vi "Scripted Autonomous.vi"   [LabVIEW 2015]
uses:
  Common Code/Change Detect Int.vi
  Robot Global Data.vi
types:
  T1 = typedef "Auton Command Cluster.ctl" = cluster{"Command ID":i32, "maxTime":dbl, "Y Distance":dbl, "Heading":dbl, "Throttle":dbl, "Async":dbl, "Velocity":dbl, "Acceleration":dbl, "To":dbl, "Condition":dbl, "Shot Type":dbl, "Left RPM":dbl, "Override RPM":i32, "Override Angle":i32, "Right RPM":dbl, "Angle":dbl, "Intake Mode":i32, "Intake Cmd":i32, "Intake O":i32, "Eject O":i32, "Angle O":i32, "Arm O":i32, "Intake Speed":dbl, "Eject Speed":dbl, "Arm Angle":dbl, "Arm Speed":dbl, "Intake?":i32, "Eject?":i32}
  T2 = typedef "Drivetrain Status Cluster.ctl" = cluster{"Modes":T3, "Y (Throttle)":dbl, "X (Steer)":dbl, "Gyro In Range?":bool, "Distance Drive Finished?":bool, "Stop Eject Lockout":bool, "Dist Drive Status":T4, "Y Target":dbl, "Heading Target":dbl, "Vision Target Aligned?":bool, "Gear":dbl, "1st Gear Time":dbl, "2nd Gear Time":dbl, "1st Gear Shifts":dbl, "2nd Gear Shifts":dbl}
  T3 = typedef "Drivetrain Modes.ctl" = enum16{"Climb", "Manual", "Ball Vision Targeting", "Goal Vision Targeting", "PID Distance Drive", "Hybrid"}
  T4 = typedef "Dist Drive Status.ctl" = cluster{"Y In Range":bool, "X In Range":bool, "Gyro In Range":bool, "Y Dist":dbl, "X Dist":dbl, "Gyro":dbl}
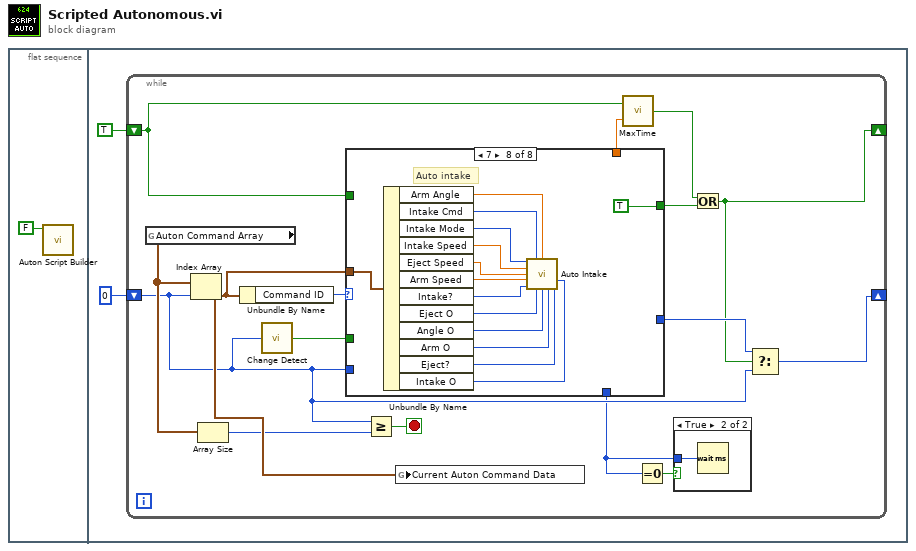
[diagram p0: block diagram]
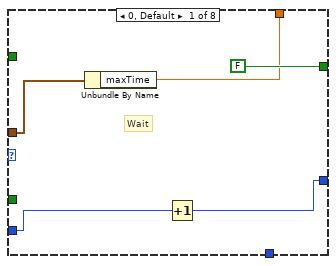
[diagram p3: hidden frame]
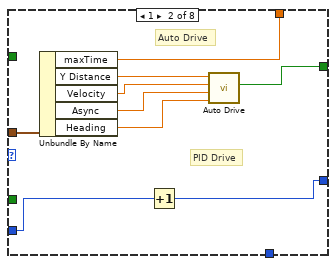
[diagram p4: hidden frame]
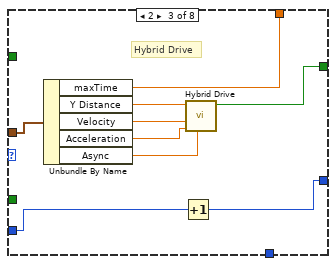
[diagram p5: hidden frame]
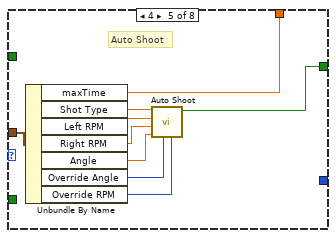
[diagram p7: hidden frame]
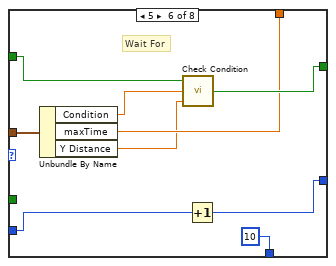
[diagram p8: hidden frame]
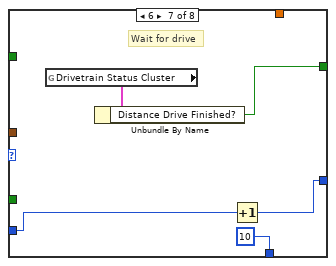
[diagram p9: hidden frame]
diagram:
  n1 = flat-sequence {
    frame #0 {
      n2 = call "Auton Script Builder.vi"("Export?"=FALSE) -> ()  [unwired: 11 in]
    }
    frame #1 {
      n3 = while {
        shift-right: [w12] -> _
        shift-left: 0 -> [w13]
        shift-right: [w9] -> _
        shift-left: TRUE -> [w6]
        stop <- w14 stop-if-true
        n4 = global read "Robot Global Data.vi" "Auton Command Array"() -> (w16:T1[])
        n5 = Index Array(array=w16, index=w13) -> (element=w19:T1)
        n6 = Array Size(array=w16) -> (size(s)=w15:i32)
        n7 = Unbundle By Name(w19) -> ("Command ID"=w18:i32)
        n8 = call-poly "Change Detect.vi"("In"=w13) -> ("Changed?"=w17:bool)
        n9 = case shown="7" w18 {
          tunnel: w13 -> [w23 w27 w36 _ _ w55 w65 _]
          tunnel: w17 -> [_ _ _ _ _ _ _ _]
          tunnel: w6 -> [_ _ _ _ _ w61 _ _]
          tunnel: [w24 w26 w35 _ _ w53 w66 _] -> w11
          tunnel: [FALSE w28 w39 _ w44 w60 w64 TRUE] -> w10
          tunnel: [w21 w33 w37 _ w45 w58 _ _] -> w7
          tunnel: w19 -> [w22 w34 w43 _ w52 w56 _ w79]
          tunnel: [_ _ _ _ _ 10 10 _] -> w5
          frame 0, Default {
            # "Wait"
            n10 = Unbundle By Name(w22) -> ("maxTime"=w21:dbl)
            n11 = Increment(x=w23) -> (x+1=w24:i32)
          }
          frame 1 {
            # "Auto Drive"
            # "PID Drive"
            n12 = Unbundle By Name(w34) -> ("maxTime"=w33:dbl, "Y Distance"=w32:dbl, "Velocity"=w31:dbl, "Async"=w30:dbl, "Heading"=w29:dbl)
            n13 = Increment(x=w27) -> (x+1=w26:i32)
            n14 = call "Auto Drive.vi"("heading"=w29, "async"=w30, "speed"=w31, "y"=w32) -> ("isFinished?"=w28:bool)  [unwired: 7 in]
          }
          frame 2 {
            # "Hybrid Drive"
            n15 = Unbundle By Name(w43) -> ("maxTime"=w37:dbl, "Y Distance"=w42:dbl, "Velocity"=w41:dbl, "Acceleration"=w40:dbl, "Async"=w38:dbl)
            n16 = Increment(x=w36) -> (x+1=w35:i32)
            n17 = call "Hybrid Drive.vi"("Async?"=w38, "Max Accel"=w40, "Max Velocity"=w41, "Distance"=w42) -> ("Finished?"=w39:bool)  [unwired: 7 in]
          }
          frame 3 {
            # "Jump"
          }
          frame 4 {
            # "Auto Shoot"
            n18 = Unbundle By Name(w52) -> ("maxTime"=w45:dbl, "Shot Type"=w51:dbl, "Left RPM"=w50:dbl, "Right RPM"=w49:dbl, "Angle"=w48:dbl, "Override Angle"=w47:i32, "Override RPM"=w46:i32)
            n19 = call "Auto Shoot.vi"("RPM Override?"=w46, "Angle Override?"=w47, "Angle"=w48, "Right RPM"=w49, "Left RPM"=w50, "Shot Type"=w51) -> ("Finished?"=w44:bool)  [unwired: 5 in]
          }
          frame 5 {
            # "Wait For"
            n20 = Unbundle By Name(w56) -> ("Condition"=w59:dbl, "maxTime"=w58:dbl, "Y Distance"=w57:dbl)
            n21 = call "Check Condition.vi"("Distance"=w57, "Condition"=w59, "Reset"=w61) -> ("Done"=w60:bool)
            n22 = Increment(x=w55) -> (x+1=w53:i32)
          }
          frame 6 {
            # "Wait for drive"
            n23 = global read "Robot Global Data.vi" "Drivetrain Status Cluster"() -> (w63:T2)
            n24 = Unbundle By Name(w63) -> ("Distance Drive Finished?"=w64:bool)
            n25 = Increment(x=w65) -> (x+1=w66:i32)
          }
          frame 7 {
            # "Auto intake"
            n26 = Unbundle By Name(w79) -> ("Arm Angle"=w78:dbl, "Intake Cmd"=w77:i32, "Intake Mode"=w76:i32, "Intake Speed"=w75:dbl, "Eject Speed"=w74:dbl, "Arm Speed"=w73:dbl, "Intake?"=w72:i32, "Eject O"=w71:i32, "Angle O"=w70:i32, "Arm O"=w69:i32, "Eject?"=w68:i32, "Intake O"=w67:i32)
            n27 = call "Auto Intake.vi"("Intake Mode ID"=w76, "Intake Command ID"=w77, "Arm Angle"=w78, "Intake Override Speed"=w75, "Eject Override Speed"=w74, "Arm Speed"=w73, "Override Intake?"=w67, "Intake?"=w72, "Override Eject?"=w71, "Override Angle?"=w70, "Override Arm?"=w69, "Eject?"=w68) -> ()  [unwired: 4 in]
          }
        }
        n28 = Greater Or Equal?(x=w13, y=w15) -> (x >= y?=w14:bool)
        n29 = global write "Robot Global Data.vi" "Current Auton Command Data"(w19) -> ()
        n30 = call "MaxTime.vi"("MaxTime"=w7, "Reset?"=w6) -> ("Finished?"=w8:bool)
        n31 = Equal To 0?(x=w5) -> (x = 0?=w4:bool)
        n32 = case shown="True" w4 {
          tunnel: w5 -> [_ w20]
          frame False {
          }
          frame True {
            n33 = Wait (ms)(milliseconds to wait=w20) -> ()  [unwired: 1 out]
          }
        }
        n34 = Or(x=w8, y=w10) -> (x .or. y?=w9:bool)
        n35 = Select(t=w11, s=w9, f=w13) -> (s? t:f=w12:i32)
      }
    }
  }
